vi "Round Log.vi"(0 "value":dbl format="%#_6p") -> (1 "upper log":dbl format="%#_6p", 2 "nearest log":dbl format="%#_6p", 3 "lower log":dbl format="%#_6p")   [LabVIEW 2020]
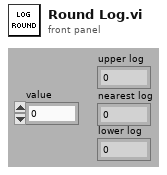
[diagram p1: front panel]
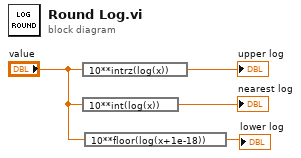
[diagram p0: block diagram]
diagram:
  n1 = expression code="10**intrz(log(x))"("value") -> (→"upper log":dbl)
  n2 = expression code="10**int(log(x))"("value") -> (→"nearest log":dbl)
  n3 = expression code="10**floor(log(x+1e-18))"("value") -> (→"lower log":dbl)
